vi "Sandbox 4 - Get Virtual Folder Structure.vi"() -> ()   [LabVIEW 2022 SP3]
panel:
  out "Project Item Names (Folders)":string[](array[string])
  out "Project Item Names (VIs)":string[](array[string])
  out "ItemIDs":string[](array[string])
  out "TypeGUIDs":string[](array[string])
  out "TypeStrings":string[](array[string])
  out "LibraryItemTypeStrings":string[](array[string])
  out "LibraryItemTypes":string[](array[string])
  out "Names":string[](array[string])
  out "Number of owned items":i32
  out "error out":errorcluster
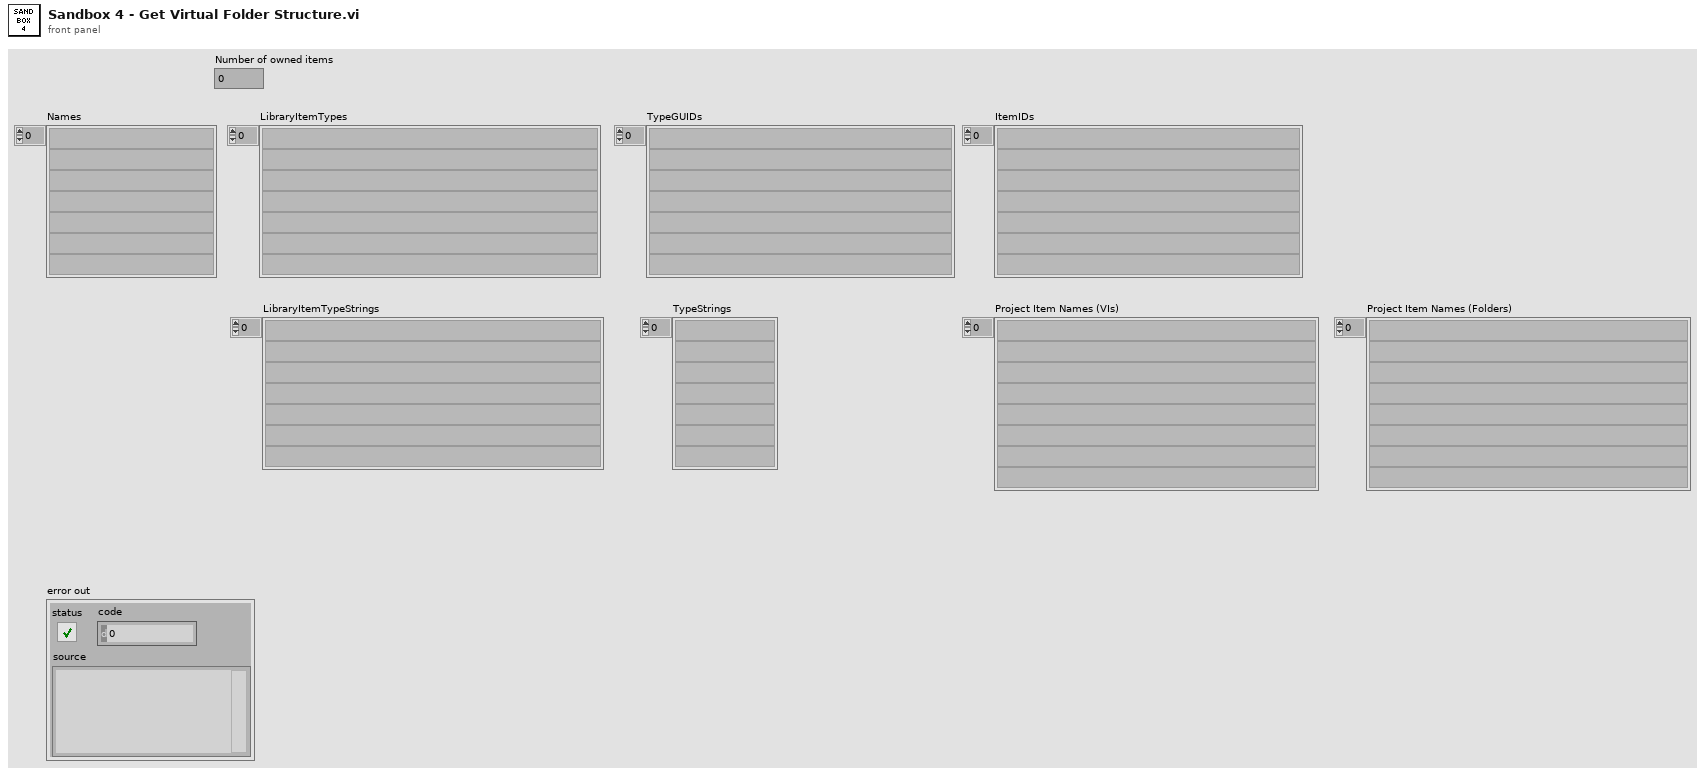
[diagram p1: front panel]
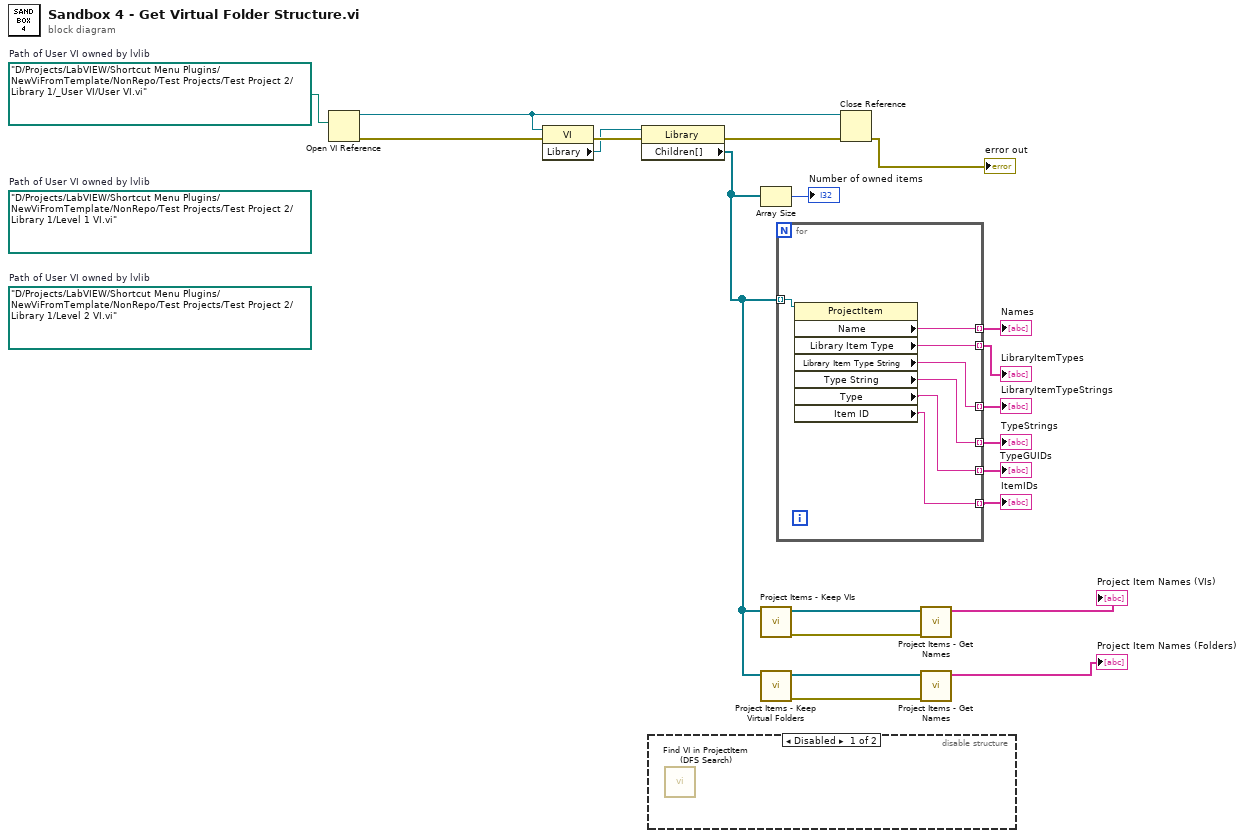
[diagram p0: block diagram]
diagram:
  (unwired) path "D:/Projects/LabVIEW/Shortcut Menu Plugins/NewViFromTemplate/NonRepo/Test Projects/Test Project 2/Library 1/Level 2 VI.vi"  # Path of User VI owned by lvlib
  (unwired) path "D:/Projects/LabVIEW/Shortcut Menu Plugins/NewViFromTemplate/NonRepo/Test Projects/Test Project 2/Library 1/Level 1 VI.vi"  # Path of User VI owned by lvlib
  w21 = path "D:/Projects/LabVIEW/Shortcut Menu Plugins/NewViFromTemplate/NonRepo/Test Projects/Test Project 2/Library 1/_User VI/User VI.vi"  # Path of User VI owned by lvlib
  n1 = Open VI Reference(vi path=w21) -> (vi reference=w17:refnum<vi>, error out=w20:errorcluster)  [unwired: 5 in]
  n2 = property class="VI"(reference=w17, error in=w20) -> (error out=w18:errorcluster, "Library"=w15:refnum<vi>)  [unwired: 1 out]
  n3 = property class="Library"(reference=w15, error in=w18) -> (error out=w16:errorcluster, "Children[]"=w4:refnum<vi>[])  [unwired: 1 out]
  n4 = disable-structure shown="Disabled" {
    frame Disabled {
      n5 = call "Find VI in ProjectItem (DFS Search).vi"() -> ()  [unwired: 10 in, 2 out]
    }
    frame Enabled {
    }
  }
  n6 = Array Size(array=w4) -> (size(s)=→"Number of owned items":i32)
  n7 = call "Project Items - Keep VIs.vi"("Project Items"=w4) -> ("Error Out"=w6:errorcluster, "Project Items (VIs)"=w7:refnum<vi>[])  [unwired: 9 in]
  n8 = call "Project Items - Keep Virtual Folders.vi"("Project Items"=w4) -> ("Error Out"=w3:errorcluster, "Project Items (Folders)"=w2:refnum<vi>[])  [unwired: 9 in]
  n9 = for {
    tunnel: w4 -> [w28] mode=indexing
    tunnel: [w27] -> w13 mode=indexing
    tunnel: [w26] -> w12 mode=indexing
    tunnel: [w25] -> w11 mode=indexing
    tunnel: [w24] -> w10 mode=indexing
    tunnel: [w23] -> w9 mode=indexing
    tunnel: [w22] -> w8 mode=indexing
    n10 = property class="ProjectItem"(reference=w28) -> ("Name"=w27:string, "Library Item Type"=w26:string, "Library Item Type String"=w25:string, "Type String"=w24:string, "Type"=w23:string, "Item ID"=w22:string)  [unwired: 1 in, 2 out]
  }
  "Names" <- w13
  "LibraryItemTypes" <- w12
  "LibraryItemTypeStrings" <- w11
  "TypeStrings" <- w10
  "TypeGUIDs" <- w9
  "ItemIDs" <- w8
  n11 = Close Reference(reference=w17, error in (no error)=w16) -> (error out=→"error out":errorcluster)
  n12 = call "Project Items - Get Names.vi"("Error In"=w6, "Project Items"=w7) -> ("Project Item Names"=→"Project Item Names (VIs)":string[])  [unwired: 8 in, 1 out]
  n13 = call "Project Items - Get Names.vi"("Error In"=w3, "Project Items"=w2) -> ("Project Item Names"=→"Project Item Names (Folders)":string[])  [unwired: 8 in, 1 out]
